vi "JSONRead.vi"(8 "error in":errorcluster, 10 "CameraController ID":string="0", 11 "file path (use dialog)":path) -> (0 "error out":errorcluster, 3 "Camera Controller Parameters":T1)   [LabVIEW 2019, in "Camera Controller.lvlib" / "Camera Controller.lvclass"]
uses:
  Camera Controller.lvclass
  TypeDef/CameraControllerParameters.ctl
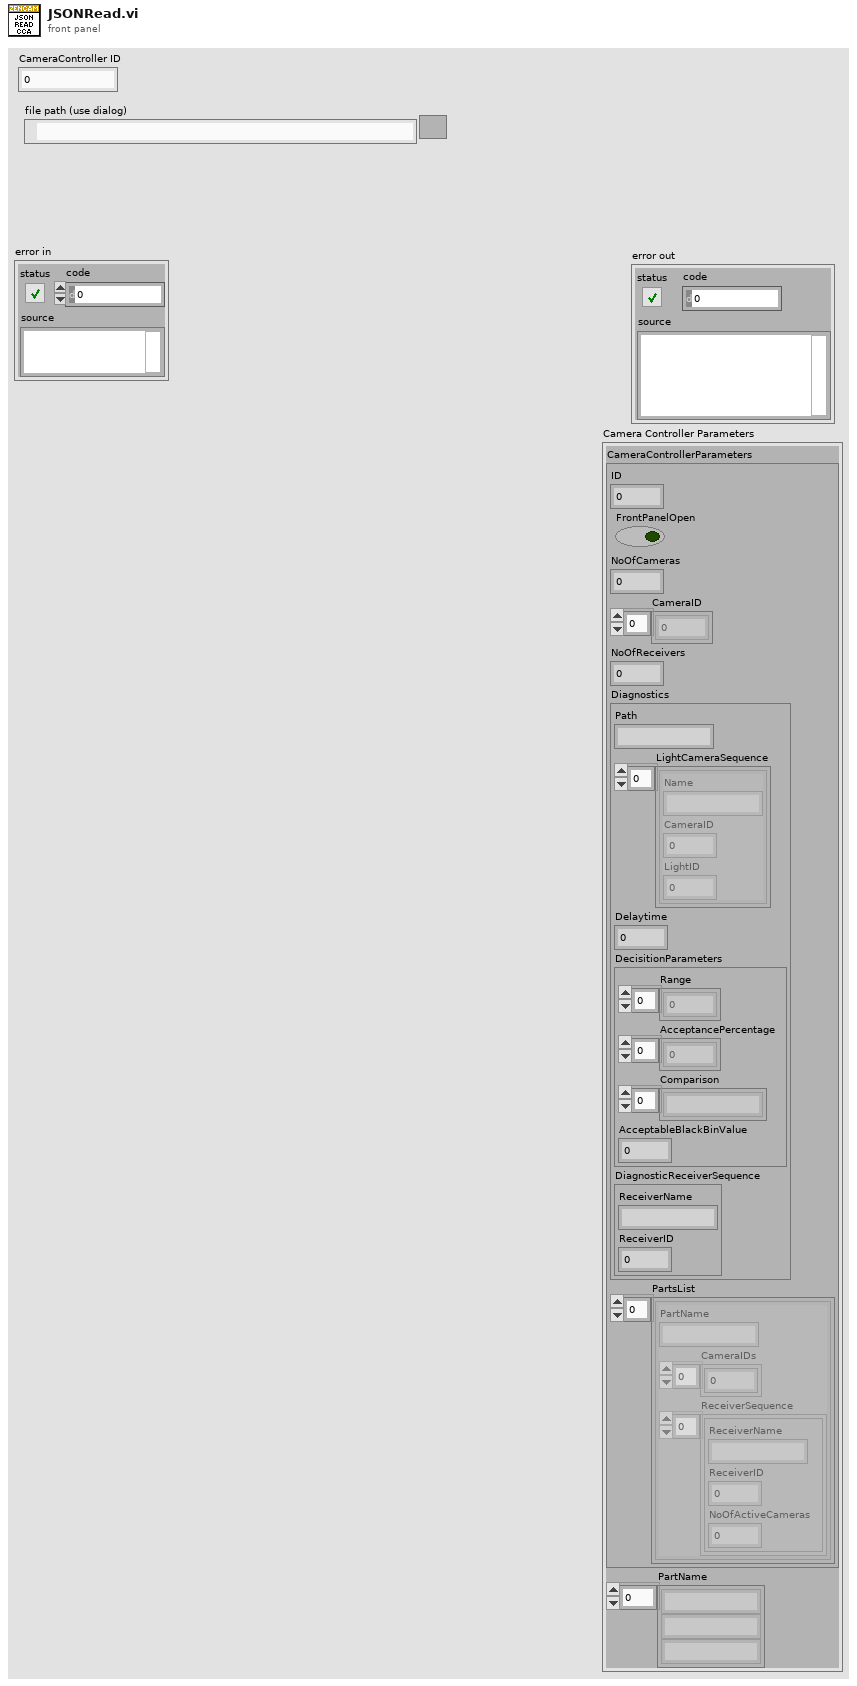
[diagram p1: front panel]
types:
  T1 = typedef "Camera Controller.lvlib/Camera Controller.lvclass/CameraControllerParameters.ctl" = cluster{"CameraControllerParameters":cluster{"ID":i32, "FrontPanelOpen":bool, "NoOfCameras":i32, "CameraID":i32[], "NoOfReceivers":i32, "Diagnostics":cluster{"Path":string, "LightCameraSequence":cluster{"Name":string, "CameraID":i32, "LightID":i32}[], "Delaytime":dbl, "DecisitionParameters":cluster{"Range":i32[], "AcceptancePercentage":i32[], "Comparison":string[], "AcceptableBlackBinValue":i32}, "DiagnosticReceiverSequence":cluster{"ReceiverName":string, "ReceiverID":i32}}, "PartsList":cluster{"PartName":string, "CameraIDs":i32[], "ReceiverSequence":cluster{"ReceiverName":string, "ReceiverID":i32, "NoOfActiveCameras":i32}[]}[]}, "PartName":string[]}
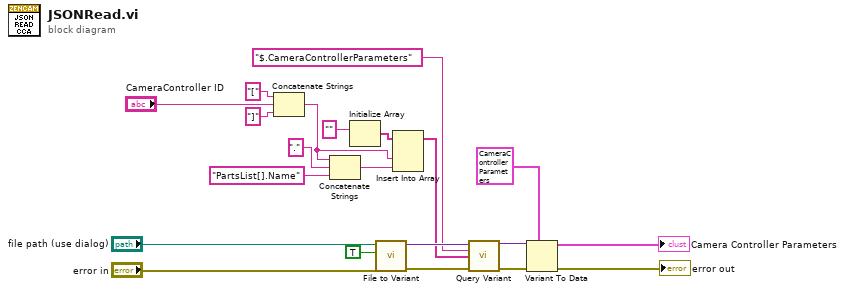
[diagram p0: block diagram]
diagram:
  n1 = Concatenate Strings("[" ("string"), "CameraController ID", "]" ("string")) -> (w16:string)
  n2 = Concatenate Strings(w16, "." ("string"), "PartsList[].Name" ("new element/subarray")) -> (w10:string)
  n3 = Initialize Array("") -> (w20:string[])  [unwired: 1 in]
  n4 = call <vilib>:"File to Variant.vi"("JSON FilePath"="file path (use dialog)", "Remove Comments?"=TRUE, "error in (no error)"="error in") -> ("JSON Variant"=w6:variant, "error out"=w5:errorcluster)  [unwired: 5 in, 1 out]
  n5 = Insert Into Array(array=w20, new element #1=w16, new element #2=w10) -> (w1:string[])  [unwired: 1 in]
  n6 = call <vilib>:"Query Variant.vi"("VCluster in"=w6, "basePath in"="$.CameraControllerParameters", "pathList"=w1, "error IO"=w5) -> ("VCluster\n out"=w3:variant, "error out"=w4:errorcluster)  [unwired: 8 in, 2 out]
  n7 = Variant To Data(error in=w4, type=T1 {"CameraControllerParameters"={"ID"=0, "FrontPanelOpen"=FALSE, "NoOfCameras"=0, "CameraID"=[], "NoOfReceivers"=0, "Diagnostics"={"Path"="", "LightCameraSequence"=[], "Delaytime"=0.0, "DecisitionParameters"={"Range"=[], "AcceptancePercentage"=[], "Comparison"=[], "AcceptableBlackBinValue"=0}, "DiagnosticReceiverSequence"={"ReceiverName"="", "ReceiverID"=0}}, "PartsList"=[]}, "PartName"=[]}, Variant=w3) -> (data=→"Camera Controller Parameters":T1, error out=→"error out":errorcluster)
